vi "BrakeReleaseAccess.vi"(0 "Operation Interface in":refnum<class "Operation Interface.lvclass">, 1 "Robot Status in":T1, 5 "error in (no error)":errorcluster) -> (14 "Operation Interface out":refnum<class "Operation Interface.lvclass">, 15 "Robot Status out":T1, 19 "error out":errorcluster)   [LabVIEW 2016, in "Operation Interface.lvclass"]
uses:
  Operation Interface.lvclass
  Robot/Universal Robot/RobotStatus.ctl
  Robot/Universal Robot/RobotMode.ctl
  Robot/Universal Robot/OperationalMode.ctl
  Robot/Universal Robot/SafetyStatus.ctl
  Operation Interface.lvclass/Operation Interface.ctl
  Robot/Universal Robot/Universal Robot.lvclass
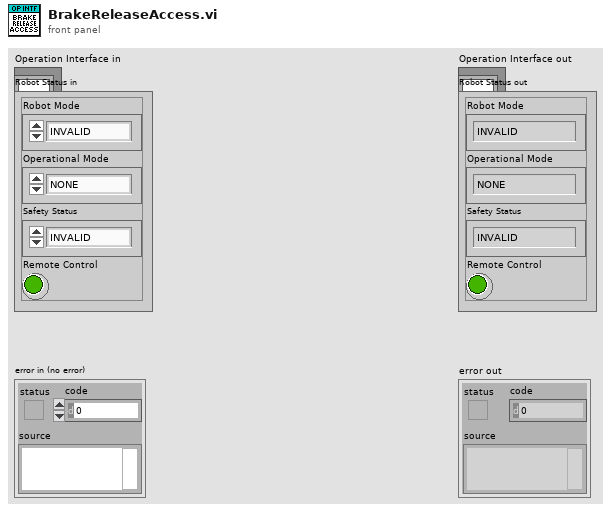
[diagram p1: front panel]
types:
  T1 = typedef "Universal Robot.lvclass/RobotStatus.ctl" = cluster{"Robot Mode":T2, "Operational Mode":T3, "Safety Status":T4, "Remote Control":bool}
  T2 = typedef "Universal Robot.lvclass/RobotMode.ctl" = enum16{"INVALID", "NO_CONTROLLER", "DISCONNECTED", "CONFIRM_SAFETY", "BOOTING", "POWER_OFF", "POWER_ON", "IDLE", "BACKDRIVE", "RUNNING"}
  T3 = typedef "Universal Robot.lvclass/OperationalMode.ctl" = enum16{"NONE", "MANUAL", "AUTOMATIC"}
  T4 = typedef "Universal Robot.lvclass/SafetyStatus.ctl" = enum16{"INVALID", "NORMAL", "REDUCED", "PROTECTIVE_STOP", "RECOVERY", "SAFEGUARD_STOP", "SYSTEM_EMERGENCY_STOP", "ROBOT_EMERGENCY_STOP", "VIOLATION", "FAULT", "AUTOMATIC_MODE_SAFEGAURD_STOP", "SYSTEM_THREE_POSITION_ENABLING_STOP"}
  T5 = enum8{"Enabled", "Disabled", "Disabled and Grayed Out"}
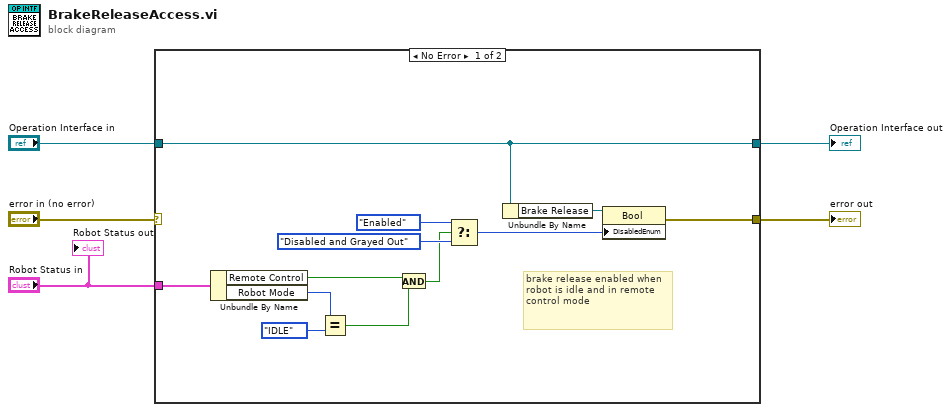
[diagram p0: block diagram]
diagram:
  n1 = case shown="No Error" "error in (no error)" {
    selector: "error in (no error)" -> [_ w19]
    tunnel: [w9 w19] -> w4
    tunnel: [w17 w18] -> w2
    tunnel: "Operation Interface in" -> [w17 w18]
    tunnel: "Robot Status in" -> [w16 _]
    frame No Error {
      # "brake release enabled when robot is idle and in remote control mode"
      n2 = Unbundle By Name(w16) -> ("Remote Control"=w8:bool, "Robot Mode"=w11:T2)
      n3 = Equal?(x=w11, y=RobotMode."IDLE" ("x")) -> (x = y?=w7:bool)
      n4 = And(x=w8, y=w7) -> (x .and. y?=w6:bool)
      n5 = Select(t=T5."Enabled" ("Disabled"), s=w6, f=T5."Disabled and Grayed Out" ("Disabled")) -> (s? t:f=w10:T5)
      n6 = Unbundle By Name(w17) -> ("Brake Release"=w13:refnum<vi>)
      n7 = property class="Bool"(reference=w13, "DisabledEnum"=w10) -> (error out=w9:errorcluster)  [unwired: 1 in, 1 out]
    }
    frame Error {
    }
  }
  "error out" <- w4
  "Operation Interface out" <- w2
  "Robot Status out" <- "Robot Status in"
